vi "Write Music Element Library.vi"(8 "error in (no error)":errorcluster, 10 "Music Element Library":refnum<class "MusicElement.lvclass">[](array[class]), 11 "MusicElementLibrary in":refnum<class "MusicElementLibrary.lvclass">) -> (0 "error out":errorcluster, 3 "MusicElementLibrary out":refnum<class "MusicElementLibrary.lvclass">)   [LabVIEW 2015, in "MusicElementLibrary.lvclass"]
uses:
  MusicElementLibrary.lvclass
  MusicElement.lvclass
  MusicElementLibrary.lvclass/MusicElementLibrary.ctl
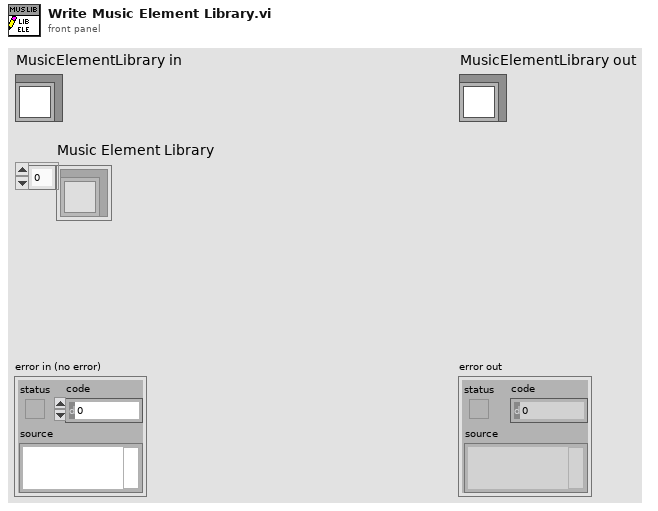
[diagram p1: front panel]
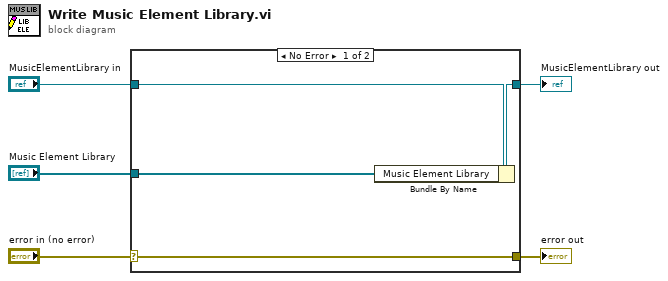
[diagram p0: block diagram]
diagram:
  n1 = case shown="No Error" "error in (no error)" {
    selector: "error in (no error)" -> [w9 w10]
    tunnel: [w9 w10] -> w4
    tunnel: [w7 w11] -> w2
    tunnel: "MusicElementLibrary in" -> [w8 w11]
    tunnel: "Music Element Library" -> [w6 _]
    frame No Error {
      n2 = Bundle By Name(cluster=w8, "Music Element Library"=w6) -> (w7:refnum<class "MusicElementLibrary.lvclass">)
    }
    frame Error {
    }
  }
  "error out" <- w4
  "MusicElementLibrary out" <- w2
